vi "NET-RX UDP Service.vi"(7 "Max Rx Byte Size":i32=10000, 8 "Module ID":i32=-1, 9 "Caller MsgQ":refnum<class "DQMH-GenNet Message Queue.lvclass">, 10 "Stop Module":refnum<user-event>, 11 "UDP Connection ID":refnum<k16>) -> ()   [LabVIEW 2014, in "GenNet-Client.lvlib"]
uses:
  GenNet-Client.lvlib
  DQMH-GenNet Message Queue.lvclass
  GenNet-Server/Stop Argument--cluster.ctl
  <vilib>/Delacor/Delacor QMH/Libraries/Message Queue_class/Delacor_lib_QMH_Message Queue.lvclass/Delacor_lib_QMH_Message Queue.ctl
  <vilib>/Delacor/Delacor QMH/Libraries/Message Queue_class/Delacor_lib_QMH_Enqueue Message (Single).vi
  GenNet Version-Safe Unflatten Variant.vi
  <vilib>/Delacor/Delacor QMH/Libraries/Message Queue_class/Delacor_lib_QMH_Message Queue.lvclass
  hse-gennet.lvlib
  GenNet-Server/GenNet-Server.lvlib
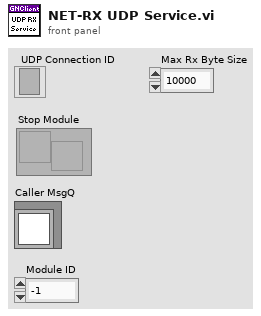
[diagram p1: front panel]
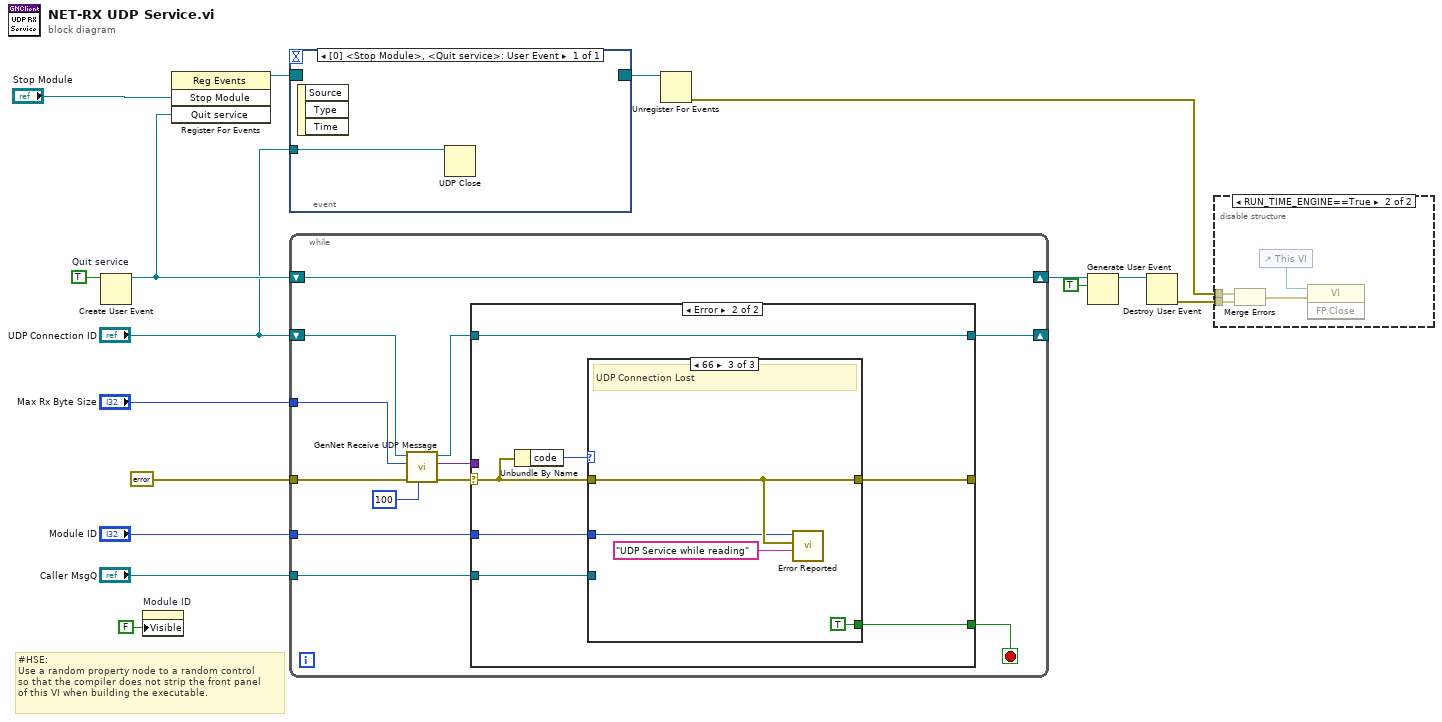
[diagram p0: block diagram]
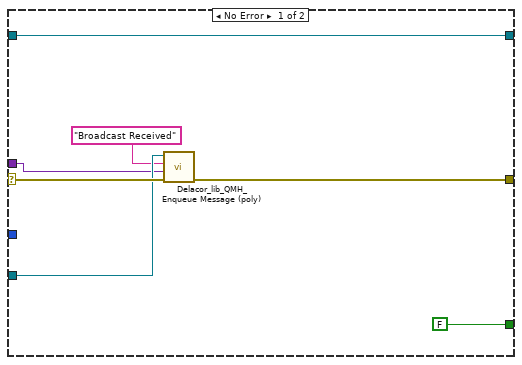
[diagram p3: hidden frame]
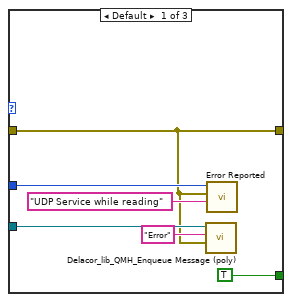
[diagram p4: hidden frame]
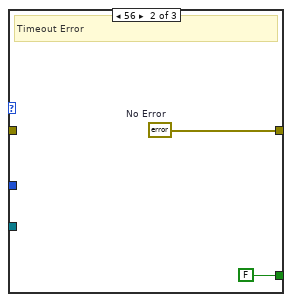
[diagram p5: hidden frame]
diagram:
  w11 = TRUE  # Quit service
  # "#HSE: \nUse a random property node to a random control \nso that the compiler does not strip the front panel \nof this VI when building the executable."
  n1 = Create User Event(user event datatype=w11) -> (user event=w12:refnum<user-event>)  [unwired: 1 in, 1 out]
  n2 = property on="Module ID" class="DigNum (strict)"("Visible"=FALSE) -> ()  [unwired: 2 in, 2 out]
  n3 = register-events("Stop Module", w12) -> (reference out=w10:refnum<event-registration>)  [unwired: 2 in, 1 out]
  n4 = event shown="[0] <Stop Module>, <Quit service>: User Event" {
    selector: w10 -> [_]
    dyn-events: [_] -> w16
    timeout: _ -> [_]
    tunnel: "UDP Connection ID" -> [w17]
    event User Event {
      n5 = event-data() -> ()  [unwired: 1 in, 3 out]
      n6 = UDP Close(connection ID=w17) -> ()  [unwired: 1 in, 2 out]
    }
  }
  n7 = while {
    shift-right: [w29] -> _
    shift-left: "UDP Connection ID" -> [w20]
    tunnel: errorcluster {"status"=FALSE, "code"=0, "source"=""} ("error out") -> [w24]
    shift-right: [w28] -> w13
    shift-left: w12 -> [w28]
    tunnel: "Module ID" -> [w26]
    tunnel: "Caller MsgQ" -> [w25]
    tunnel: "Max Rx Byte Size" -> [w18]
    stop <- w27 stop-if-true
    n8 = call "GenNet Receive UDP Message.vi"("timeout [ms]"=100, "error in (no error)"=w24, "Max Byte Size"=w18, "UDP Network Connection in"=w20) -> ("error out"=w23:errorcluster, "Message Data"=w22:variant, "UDP Network Connection out"=w21:refnum<k16>)  [unwired: 5 in]
    n9 = case shown="Error" w23 {
      selector: w23 -> [w35 w41]
      tunnel: w21 -> [w33 w39]
      tunnel: [w33 w39] -> w29
      tunnel: [FALSE w38] -> w27
      tunnel: w26 -> [_ w40]
      tunnel: w25 -> [w34 w42]
      tunnel: w22 -> [w31 _]
      tunnel: [w32 w37] -> _
      frame No Error {
        n10 = call-poly <vilib>:"Delacor_lib_QMH_Enqueue Message (poly).vi"("error in (no error)"=w35, "Message Data"=w31, "Message"="Broadcast Received", "Message Queue in"=w34) -> ("error out"=w32:errorcluster)  [unwired: 6 in, 1 out]
      }
      frame Error {
        n11 = Unbundle By Name(w41) -> ("code"=w43:i32)
        n12 = case shown="66" w43 {
          tunnel: w42 -> [w48 _ _]
          tunnel: w41 -> [w44 _ w55]
          tunnel: w40 -> [w47 _ w53]
          tunnel: [w44 w50 w55] -> w37
          tunnel: [TRUE FALSE TRUE] -> w38
          frame Default {
            n13 = call-poly <vilib>:"Delacor_lib_QMH_Enqueue Message (poly).vi"("Message Data"=w44, "Message"="Error", "Message Queue in"=w48) -> ()  [unwired: 7 in, 2 out]
            n14 = call "Error Reported.vi"("Additional Information"="UDP Service while reading", "Error"=w44, "Module ID"=w47) -> ()  [unwired: 8 in, 1 out]
          }
          frame 56 {
            w50 = errorcluster {"status"=FALSE, "code"=0, "source"=""}  # No Error
            # "Timeout Error"
          }
          frame 66 {
            # "UDP Connection Lost"
            n15 = call "Error Reported.vi"("Additional Information"="UDP Service while reading", "Error"=w55, "Module ID"=w53) -> ()  [unwired: 8 in, 1 out]
          }
        }
      }
    }
  }
  n16 = Unregister For Events(event registration refnum=w16) -> (error out=w4:errorcluster)  [unwired: 1 in]
  n17 = Generate User Event(user event=w13, event data cluster=TRUE ("event data")) -> (user event out=w15:refnum<user-event>)  [unwired: 2 in, 1 out]
  n18 = Destroy User Event(user event=w15) -> (error out=w5:errorcluster)  [unwired: 1 in]
  n19 = disable-structure shown="RUN_TIME_ENGINE==True" {
    disable-tunnel: w5 -> [_ w57]
    disable-tunnel: w4 -> [_ w56]
    frame condition #0 (active) {
    }
    frame condition #1 {
      n20 = Merge Errors(w56, w57) -> (w58:errorcluster)
      n21 = control-ref of="This VI"() -> (w59:refnum<vi>)
      n22 = invoke class="VI" method="FP.Close"(reference=w59, error in=w58) -> ()  [unwired: 1 in, 3 out]
    }
  }
